vi "ValidateLogPath.vi"(8 "error in (no error)":errorcluster, 11 "MassCompile in":refnum<class "MassCompile.lvclass">) -> (0 "error out":errorcluster, 3 "MassCompile out":refnum<class "MassCompile.lvclass">)   [LabVIEW 2014, in "MassCompile.lvclass"]
uses:
  MassCompile.lvclass
  MassCompile.lvclass/MassCompile.ctl
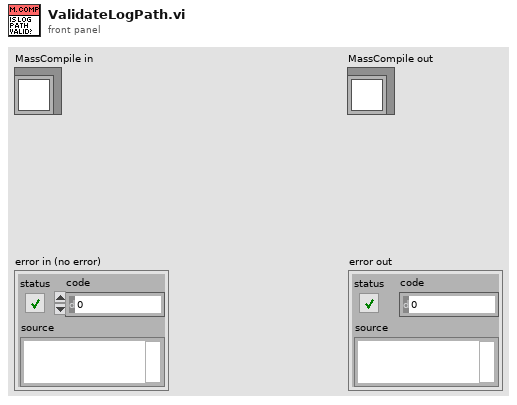
[diagram p1: front panel]
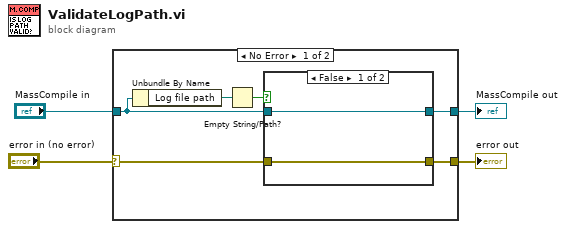
[diagram p0: block diagram]
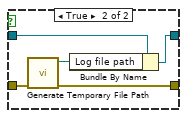
[diagram p2: hidden frame]
diagram:
  n1 = case shown="No Error" "error in (no error)" {
    selector: "error in (no error)" -> [w5 w18]
    tunnel: [w10 w18] -> w4
    tunnel: [w9 w19] -> w3
    tunnel: "MassCompile in" -> [w7 w19]
    frame No Error {
      n2 = Unbundle By Name(w7) -> ("Log file path"=w6:path)
      n3 = Empty String/Path?(string/path=w6) -> (empty?=w8:bool)
      n4 = case shown="False" w8 {
        tunnel: w7 -> [w12 w17]
        tunnel: [w12 w16] -> w9
        tunnel: w5 -> [w11 w14]
        tunnel: [w11 w13] -> w10
        frame False {
        }
        frame True {
          n5 = call <vilib>:"Generate Temporary File Path.vi"("error in (no error)"=w14) -> ("error out"=w13:errorcluster, "Unique Temporary File Path"=w15:path)  [unwired: 9 in]
          n6 = Bundle By Name(cluster=w17, "Log file path"=w15) -> (w16:refnum<class "MassCompile.lvclass">)
        }
      }
    }
    frame Error {
    }
  }
  "error out" <- w4
  "MassCompile out" <- w3
